vi "GetMeasureOn.vi"(8 "error in (no error)":errorcluster) -> (0 "error out":errorcluster, 2 "Measure On 2":bool, 3 "Measure On 1":bool)   [LabVIEW 2015, in "ESLSCDLL.lvlib"]
uses:
  ESLSCDLL.lvlib
  Globals.vi
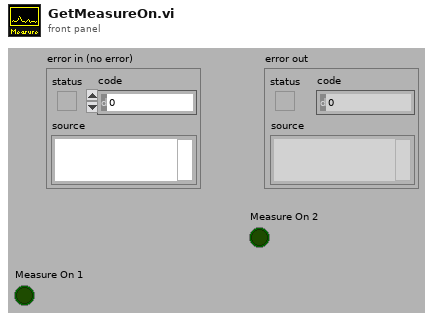
[diagram p1: front panel]
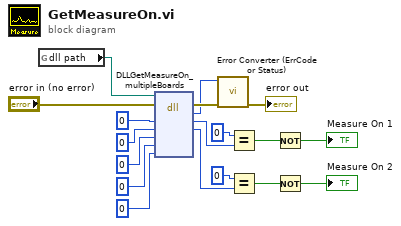
[diagram p0: block diagram]
diagram:
  n1 = global read "Globals.vi" "dll path"() -> (w1:path)
  n2 = dll-call lib="C:/ENTW/PCIE/LV64/board.vis/ESLSCDLL.dll" fn="DLLGetMeasureOn_multipleBoards" ("lwlscdll.dll:DLLWriteLongS0")(path in=w1, error in="error in (no error)", "measureOn0"=u8 0 ("measureOn"), "measureOn1"=u8 0, "measureOn2"=u8 0, "measureOn3"=u8 0, "measureOn4"=u8 0) -> (error out=w9:errorcluster, "es_status_codes"=w8:i32, "measureOn0"=w15:u8, "measureOn1"=w5:u8)  [unwired: 4 in, 1 out]
  n3 = call "Error Converter (ErrCode or Status).vi"("error in (no error)"=w9, "error code"=w8) -> ("error out"=→"error out":errorcluster)  [unwired: 9 in]
  n4 = Equal?(x=u8 0, y=w15) -> (x = y?=w17:bool)
  n5 = Equal?(x=u8 0, y=w5) -> (x = y?=w13:bool)
  n6 = Not(x=w17) -> (.not. x?=→"Measure On 1":bool)
  n7 = Not(x=w13) -> (.not. x?=→"Measure On 2":bool)
